vi "Refresh Frame Settings.vi"(8 "error in (no error)":errorcluster, 11 "Device Item Ref in":T1 format="%.0x") -> (0 "error out":errorcluster)   [LabVIEW 2015, in "Protection and Rolling Counter Addon System Explorer.lvlib"]
uses:
  Protection and Rolling Counter Addon System Explorer.lvlib
  <vilib>/NI Veristand/Custom Device API/Custom Device Item Ref.ctl
  <vilib>/NI Veristand/Custom Device Tools/Custom Device Utility Library/Search Direction.ctl
  Shared/SubVIs/GUID Lookup.vi
  <vilib>/NI Veristand/Custom Device Tools/Custom Device Utility Library/NI VeriStand - Search for Item by GUID.vi
  <vilib>/NI Veristand/Custom Device Tools/Custom Device Utility Library/NI VeriStand - Search for All Items by GUID.vi
  Shared/Protection and Rolling Counter Addon Shared.lvlib
  <vilib>/NI Veristand/Custom Device Tools/Custom Device Utility Library/Custom Device Utility Library.lvlib
  <vilib>/NI Veristand/Custom Device API/Custom Device API.lvlib
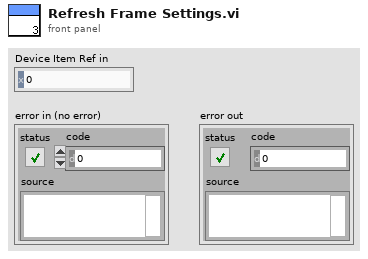
[diagram p1: front panel]
types:
  T1 = typedef "Custom Device API.lvlib/Custom Device Item Ref.ctl" = u64
  T2 = typedef "Custom Device Utility Library.lvlib/Search Direction.ctl" = enum16{"Down", "Up"}
  T3 = typedef "Protection and Rolling Counter Addon Shared.lvlib/FrameConfiguration.ctl" = cluster{"Input Channels":T4[], "Frame Rate":dbl, "Rolling Counter Count":dbl, "PCL Count":u64, "Max Count":dbl, "Frame ID":u32, "Rolling Counter":T4, "CRC":T4, "Frame Name":string, "Cluster":string, "Database":string, "Protection Type":T5}
  T4 = typedef "Protection and Rolling Counter Addon Shared.lvlib/InputChannelConfiguration.ctl" = cluster{"Start Bit":i32, "Name":string, "Node Path":string, "Number of bits":i32, "Scale":dbl, "Offset":dbl, "Data Type":u32}
  T5 = typedef "Protection and Rolling Counter Addon Shared.lvlib/Protection Type.ctl" = enum16{"Checksum", "CRC", "None (Counter Only)", "CGEA Checksum"}
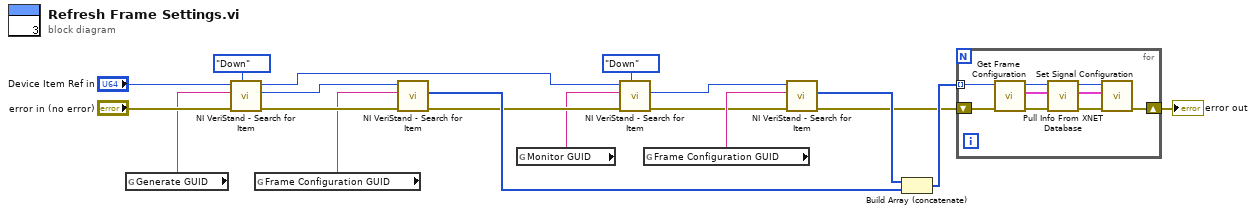
[diagram p0: block diagram]
diagram:
  n1 = global read "GUID Lookup.vi" "Generate GUID"() -> (w4:string)
  n2 = call-poly <vilib>:"NI VeriStand - Search for Item.vi"("Direction (Down)"=Search_Direction."Down", "error in"="error in (no error)", "Item GUID"=w4, "Section Ref in"="Device Item Ref in") -> ("error out"=w2:errorcluster, "Item Ref"=w3:T1, "Section Ref out"=w14:T1)  [unwired: 4 in, 1 out]
  n3 = global read "GUID Lookup.vi" "Frame Configuration GUID"() -> (w1:string)
  n4 = call-poly <vilib>:"NI VeriStand - Search for Item.vi"("error in"=w2, "Item GUID"=w1, "Section Ref in"=w3) -> ("error out"=w16:errorcluster, "Item Refs"=w17:T1[])  [unwired: 5 in, 2 out]
  n5 = global read "GUID Lookup.vi" "Monitor GUID"() -> (w9:string)
  n6 = call-poly <vilib>:"NI VeriStand - Search for Item.vi"("Direction (Down)"=Search_Direction."Down", "error in"=w16, "Item GUID"=w9, "Section Ref in"=w14) -> ("error out"=w11:errorcluster, "Item Ref"=w10:T1)  [unwired: 4 in, 2 out]
  n7 = global read "GUID Lookup.vi" "Frame Configuration GUID"() -> (w12:string)
  n8 = call-poly <vilib>:"NI VeriStand - Search for Item.vi"("error in"=w11, "Item GUID"=w12, "Section Ref in"=w10) -> ("error out"=w13:errorcluster, "Item Refs"=w18:T1[])  [unwired: 5 in, 2 out]
  n9 = Build Array (concatenate)(w18, w17) -> (w19:T1[])
  n10 = for {
    shift-right: [w20] -> w15
    shift-left: w13 -> [w22]
    tunnel: w19 -> [w21] mode=indexing
    n11 = call "Get Frame Configuration.vi"("error in"=w22, "Parent Ref"=w21) -> ("error out"=w27:errorcluster, "Selected Channels"=w25:T3, "Parent Ref Out"=w26:T1)  [unwired: 7 in]
    n12 = call "Pull Info From XNET Database.vi"("error in"=w27, "Frame Configuration"=w25, "Parent Ref"=w26) -> ("error out"=w28:errorcluster, "Frame Configuration"=w23:T3, "Item Ref out"=w24:T1)  [unwired: 6 in]
    n13 = call "Set Signal Configuration.vi"("error in"=w28, "Selected Channels"=w23, "Parent Ref"=w24) -> ("error out"=w20:errorcluster)  [unwired: 7 in, 1 out]
  }
  "error out" <- w15
